vi "Launch Interlock Chain Actor.vi"(8 "error in (no error)":errorcluster, 11 "Interlock Chain in":refnum<class "Interlock Chain.lvclass">) -> (0 "error out":errorcluster, 2 "Actor's Enqueuer":refnum<class "Message Enqueuer.lvclass">, 3 "Interlock Chain out":refnum<class "Interlock Chain.lvclass">)   [LabVIEW 2015, in "Interlocks.lvlib" / "Interlock Chain.lvclass"]
uses:
  Interlock Chain.lvclass
  <vilib>/ActorFramework/Message Enqueuer/Message Enqueuer.lvclass
  <vilib>/ActorFramework/Actor/Actor.lvclass
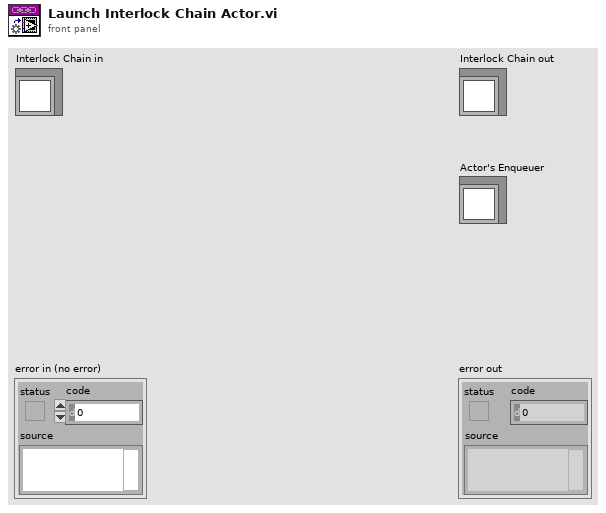
[diagram p1: front panel]
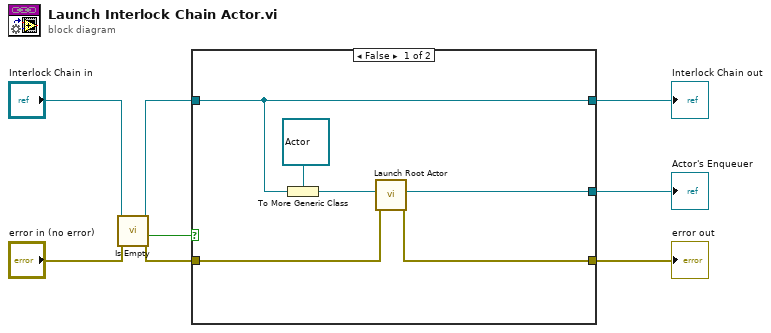
[diagram p0: block diagram]
diagram:
  n1 = call "Is Empty.vi"("error in (no error)"="error in (no error)", "Interlock Chain in"="Interlock Chain in") -> ("error out"=w4:errorcluster, "Is Empty?"=w6:bool, "Interlock Chain out"=w2:refnum<class "Interlock Chain.lvclass">)  [unwired: 7 in]
  n2 = case shown="False" w6 {
    tunnel: w4 -> [w14 w15]
    tunnel: [w13 w15] -> w5
    tunnel: w2 -> [w11 w16]
    tunnel: [w11 w16] -> w3
    tunnel: [w12 _] -> w1
    frame False {
      n3 = To More Generic Class(target class=refnum<class "Actor.lvclass"> refnum ("Actor"), reference=w11) -> (generic class reference=w9:refnum<class "Actor.lvclass">)
      n4 = call <vilib>:"Launch Root Actor.vi"("error in (no error)"=w14, "Actor"=w9) -> ("error out"=w13:errorcluster, "Actor's Enqueuer"=w12:refnum<class "Message Enqueuer.lvclass">)  [unwired: 8 in]
    }
    frame True {
    }
  }
  "error out" <- w5
  "Interlock Chain out" <- w3
  "Actor's Enqueuer" <- w1
